vi "Temprature Shift Madule Based on LMTD   main.vi"(2 "R\nRatio of Delta T down  to Delta T up":dbl, 3 "LMTD":dbl[unit], 4 "T_AD\nEvaporator Inlet cold Air Temprature":dbl[unit], 5 "T_WU\nEvaporator Inlet Hot \nWater Temprature":dbl[unit]) -> (0 "T_WD\nEvaporator Cold Outlet Water Temprature":dbl[unit], 1 "T_AU\nEvaporator Hot and Humaid Outlet \nAir Temprature":dbl[unit])   [LabVIEW 2018]
panel:
  out "T_AD\nEvaporator Inlet cold Air Temprature":dbl(slide) scale=30.0..40.0
  out "T_WD\nEvaporator Cold Outlet Water Temprature":dbl[unit](slide) scale=30.0..40.0
  out "T_WU\nEvaporator Inlet Hot \nWater Temprature":dbl[unit](slide) scale=30.0..40.0
  out "T_AU\nEvaporator Hot and Humaid Outlet \nAir Temprature":dbl[unit](slide) scale=30.0..40.0
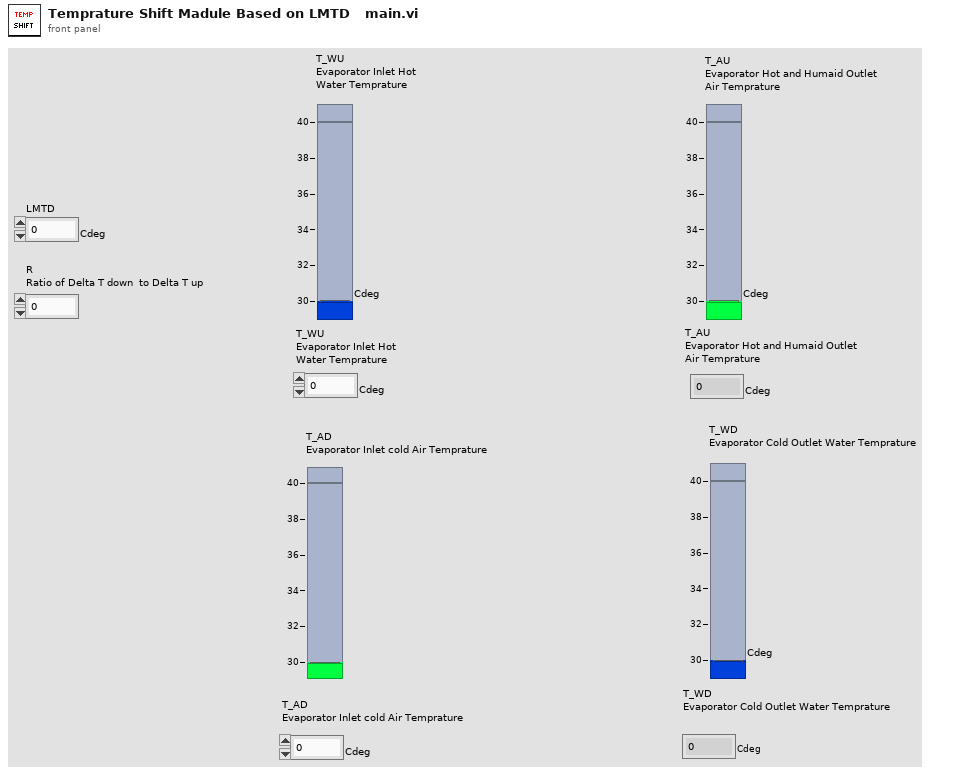
[diagram p1: front panel]
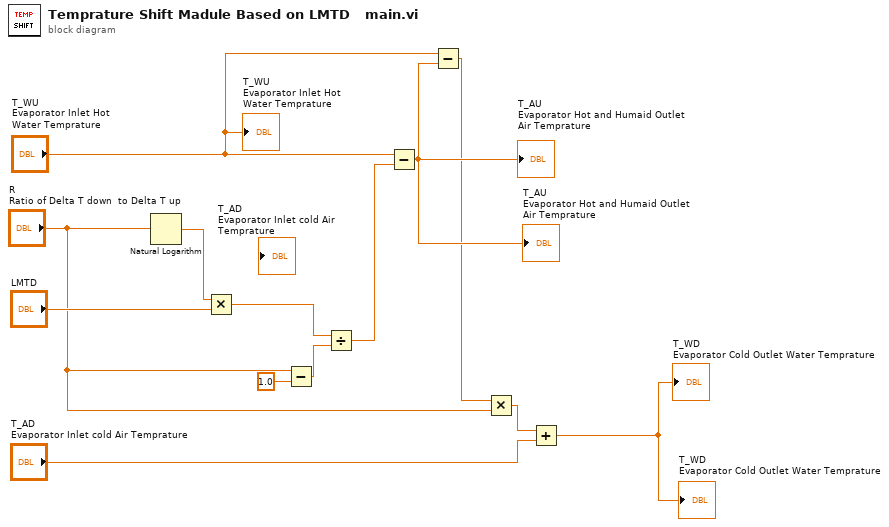
[diagram p0: block diagram]
diagram:
  n1 = Natural Logarithm(1:"R\nRatio of Delta T down  to Delta T up") -> (0:w12:dbl)
  n2 = Multiply(x=w12, y="LMTD") -> (x*y=w10:dbl[unit])
  n3 = Subtract(x="R\nRatio of Delta T down  to Delta T up", y=1.0) -> (x-y=w9:dbl)
  n4 = Divide(x=w10, y=w9) -> (x/y=w8:dbl[unit])
  n5 = Subtract(x="T_WU\nEvaporator Inlet Hot \nWater Temprature", y=w8) -> (x-y=w7:dbl[unit])
  "T_AU\nEvaporator Hot and Humaid Outlet \nAir Temprature" <- w7
  "T_AU\nEvaporator Hot and Humaid Outlet \nAir Temprature" <- w7
  n6 = Subtract(x="T_WU\nEvaporator Inlet Hot \nWater Temprature", y=w7) -> (x-y=w4:dbl[unit])
  n7 = Multiply(x=w4, y="R\nRatio of Delta T down  to Delta T up") -> (x*y=w3:dbl[unit])
  n8 = Add(x=w3, y="T_AD\nEvaporator Inlet cold Air Temprature") -> (x+y=→"T_WD\nEvaporator Cold Outlet Water Temprature" →"T_WD\nEvaporator Cold Outlet Water Temprature":dbl[unit])
  "T_WU\nEvaporator Inlet Hot \nWater Temprature" <- "T_WU\nEvaporator Inlet Hot \nWater Temprature"
